vi "p02 Integer Math.vi"() -> ()   [LabVIEW 2025]
uses:
  <vilib>/rvi/Emulation/niFpgaGetClockAttributes.vi
  <vilib>/rvi/Emulation/niFpgaSctlEmulationGetInTimedLoop.vi
  <vilib>/rvi/Emulation/niFpgaEmulationReportErrorSimple.vi
  <vilib>/rvi/eio/common/nirviEmuTemplateMethod_errors.vi
  <vilib>/rvi/Emulation/niFpgaCriticalErrorInLSC.vi
  <vilib>/eio/EIONode/EIONode.xnode
panel:
  out "Scaled":i16
  in  "n":i32=-14
  in  "y":i16=11500
  out "Connector1/AI0":i16
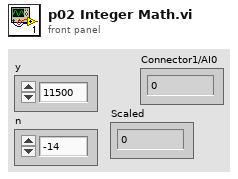
[diagram p1: front panel]
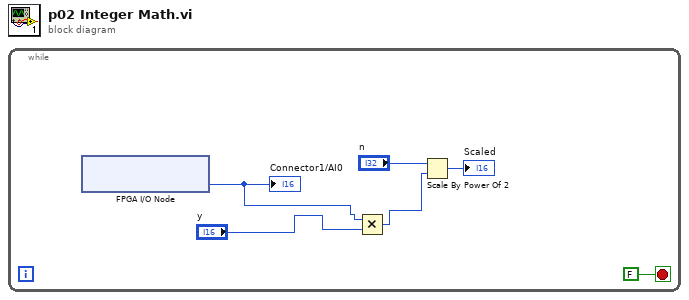
[diagram p0: block diagram]
diagram:
  n1 = while {
    stop <- FALSE stop-if-true
    n2 = xnode "FPGA I/O Node"() -> ("Connector1/AI0"=w2:i16)  [unwired: 1 in, 1 out]
    "Connector1/AI0" <- w2
    n3 = Multiply(x=w2, y="y") -> (x*y=w3:i16)
    n4 = Scale By Power Of 2(n="n", x=w3) -> (x*2^n=→"Scaled":i16)
  }
